vi "Address Pointer.vi"(1 "Register":T1(ring)) -> (0 "Pointer Register":u8[](array[numeric]))   [LabVIEW 2021]
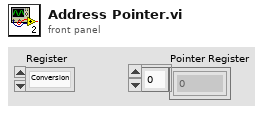
[diagram p1: front panel]
types:
  T1 = enum16{"Conversion", "Config", "LoThres", "HiThres"}
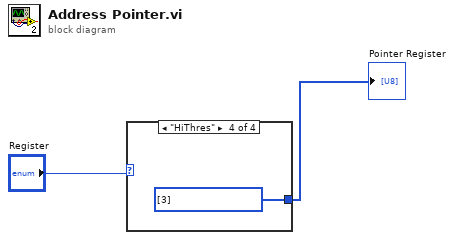
[diagram p0: block diagram]
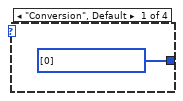
[diagram p2: hidden frame]
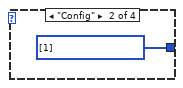
[diagram p3: hidden frame]
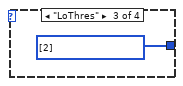
[diagram p4: hidden frame]
diagram:
  n1 = case shown="\"HiThres\"" "Register" {
    tunnel: [u8[] [0] ("Bytes to Write") u8[] [1] ("Bytes to Write") u8[] [2] ("Bytes to Write") u8[] [3] ("Bytes to Write")] -> w2
    frame "Conversion", Default {
    }
    frame "Config" {
    }
    frame "LoThres" {
    }
    frame "HiThres" {
    }
  }
  "Pointer Register" <- w2
